vi "reallocate_channel_buffers.vi"(8 "error in (no error)":errorcluster, 10 "new size":i32, 11 "ImageAssemblerDL090211Scaffold in":refnum<class "ImageAssemblerDL090211Scaffold.lvclass">) -> (0 "error out":errorcluster, 3 "ImageAssemblerDL090211Scaffold out":refnum<class "ImageAssemblerDL090211Scaffold.lvclass">)   [LabVIEW 2010, in "ImageAssemblerDL090211Scaffold.lvclass"]
uses:
  ImageAssemblerDL090211Scaffold.lvclass
  common/classes/Image/Image/Image.lvclass
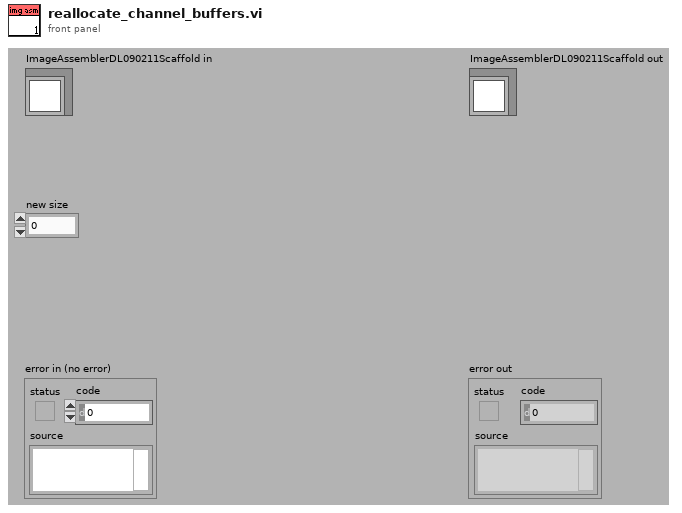
[diagram p1: front panel]
types:
  T1 = typedef "Image Type" = u32
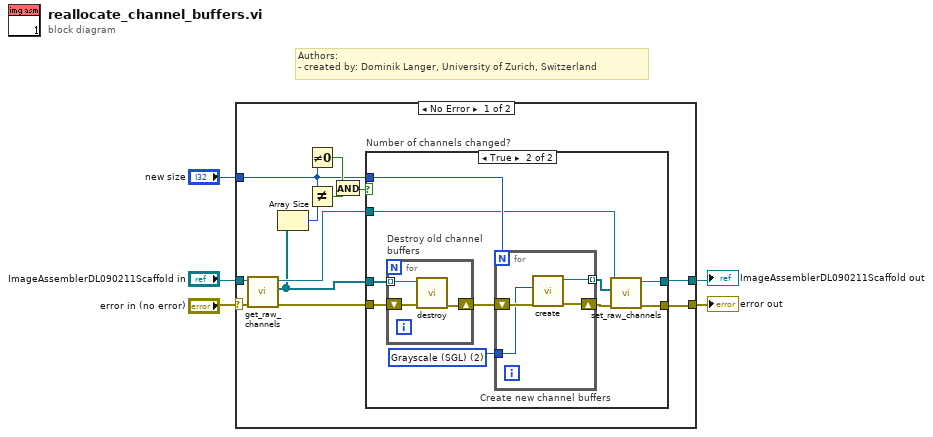
[diagram p0: block diagram]
diagram:
  # "Authors: \n- created by: Dominik Langer, University of Zurich, Switzerland"
  n1 = case shown="No Error" "error in (no error)" {
    selector: "error in (no error)" -> [w7 w38]
    tunnel: [w10 w38] -> w5
    tunnel: [w9 w37] -> w4
    tunnel: "ImageAssemblerDL090211Scaffold in" -> [w6 w37]
    tunnel: "new size" -> [w8 _]
    frame No Error {
      n2 = call-dynamic "get_raw_channels.vi"("error in (no error)"=w7, "DL090211ImageAssemblerScaffold.lvclass in"=w6) -> ("error out"=w16:errorcluster, "raw channels"=w14:refnum<class "Image.lvclass">[], "DL090211ImageAssemblerScaffold.lvclass out"=w15:refnum<class "ImageAssemblerDL090211Scaffold.lvclass">)  [unwired: 7 in]
      n3 = Array Size(array=w14) -> (size(s)=w17:i32)
      n4 = Not Equal To 0?(x=w8) -> (x != 0?=w12:bool)
      n5 = Not Equal?(x=w8, y=w17) -> (x != y?=w13:bool)
      n6 = And(x=w12, y=w13) -> (x .and. y?=w11:bool)
      n7 = case "Number of channels changed?" shown="True" w11 {
        tunnel: w16 -> [w18 w24]
        tunnel: w15 -> [w19 w20]
        tunnel: [w19 w26] -> w9
        tunnel: [w18 w25] -> w10
        tunnel: w14 -> [_ w23]
        tunnel: w8 -> [_ w21]
        frame False {
        }
        frame True {
          w27 = T1 2 items=["Grayscale (U8)", "Grayscale (I16)", "Grayscale (SGL)", "Complex (CSG)", "RGB (U32)", "HSL (U32)", "RGB (U64)", "Grayscale (U16)"] ("Image Type")
          n8 = for "Destroy old channel buffers" {
            shift-right: [w30] -> w22
            shift-left: w24 -> [w32]
            tunnel: w23 -> [w31] mode=indexing
            n9 = call-dynamic "destroy.vi"("error in (no error)"=w32, "Image in"=w31) -> ("error out"=w30:errorcluster)  [unwired: 8 in, 1 out]
          }
          n10 = for "Create new channel buffers" {
            N: w21 -> [_]
            shift-right: [w35] -> w29
            shift-left: w22 -> [w36]
            tunnel: [w34] -> w28 mode=indexing
            tunnel: w27 -> [w33]
            n11 = call "create.vi"("error in (no error)"=w36, "Image Type"=w33) -> ("error out"=w35:errorcluster, "Image out"=w34:refnum<class "Image.lvclass">)  [unwired: 2 in, 6 out]
          }
          n12 = call "set_raw_channels.vi"("error in (no error)"=w29, "raw channels"=w28, "DL090211ImageAssemblerScaffold.lvclass in"=w20) -> ("error out"=w25:errorcluster, "DL090211ImageAssemblerScaffold.lvclass out"=w26:refnum<class "ImageAssemblerDL090211Scaffold.lvclass">)  [unwired: 7 out]
        }
      }
    }
    frame Error {
    }
  }
  "error out" <- w5
  "ImageAssemblerDL090211Scaffold out" <- w4
